vi "Car Wash Cycle.vi"(4 "Finish Message":string, 6 "Start Message":string, 7 "Time (ms)":u32=5000, 9 "Indicator":refnum<class "Abs_Boolean.lvclass">, 10 "Option":refnum<class "Abs_Boolean.lvclass">, 11 "EventLog":refnum<class "Event_TextLog.lvclass">) -> (3 "bt_Node out":refnum<class "bt_Node.lvclass">)   [LabVIEW 2021, in "Car Wash Support.lvlib"]
uses:
  Car Wash Support.lvlib
  <vilib>/TSA/Event Log/Event_TextLog/Event_TextLog.lvclass
  C:/Program Files (x86)/National Instruments/LabVIEW 2021/vi.lib/TSA/Event Log/abs_EventLog/abs_EventLog.lvclass
  <vilib>/TSA/Abstract Data Classes/Abs_Types/Boolean/Abs_Boolean.lvclass
  C:/Program Files (x86)/National Instruments/LabVIEW 2021/vi.lib/TSA/Abstract Data Classes/Abs_Types/Value/Abs_Value.lvclass
  C:/Program Files (x86)/National Instruments/LabVIEW 2021/vi.lib/TSA/Abstract Data Classes/Abs_Types/Type/Abs_Type.lvclass
  Support/Nodes/abs_Node/bt_Node.lvclass
  Support/Nodes/Leaves/abs_Type Leaf/abs_Type Leaf.lvclass/abs_Type Leaf.ctl
  Support/Nodes/Leaves/abs_Type Leaf/Properties/Write Value Class.vi
  Support/Nodes/Leaves/Test Boolean/Test Abs_Boolean.lvclass
  C:/Users/timst/Documents/Repositories/LV_Behaviour_Tree/Source/Support/Nodes/abs_Node/bt_Node.lvclass
  C:/Users/timst/Documents/Repositories/LV_Behaviour_Tree/Source/Support/Nodes/Leaves/abs_Type Leaf/abs_Type Leaf.lvclass
  Support/Nodes/Leaves/Log/bt_Log.lvclass
  <vilib>/TSA/Abstract Data Classes/Constants/Support/Bool/Bool.vi
  <vilib>/TSA/Abstract Data Classes/Constants/Support/Str/Str.vi
  Support/Poly/Log/Log_StringClass.vi
  BT.lvlib
  <vilib>/TSA/Abstract Data Classes/Constants/Support/Bool/Const_Bool.lvclass
  <vilib>/TSA/Abstract Data Classes/Constants/Support/Str/Const_Str.lvclass
  C:/Program Files (x86)/National Instruments/LabVIEW 2021/vi.lib/TSA/Event Log/Event_TextLog/Event_TextLog.lvclass
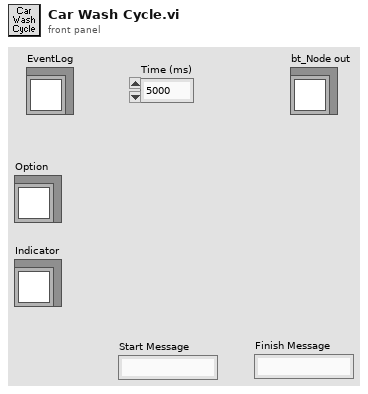
[diagram p1: front panel]
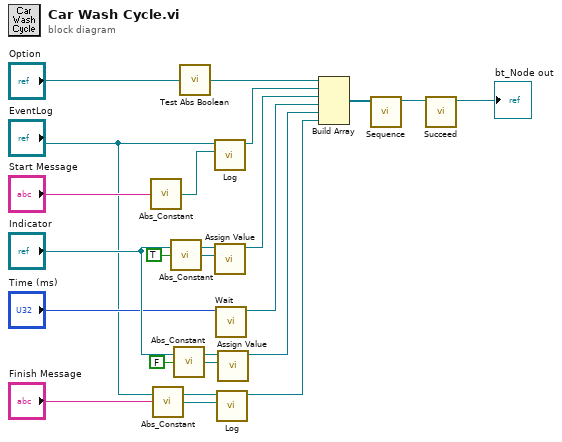
[diagram p0: block diagram]
diagram:
  n1 = call-poly <vilib>:"Abs_Constant.vi"("String"="Start Message") -> ("Abs_String.lvclass"=w16:refnum<class "Abs_String.lvclass">)  [unwired: 4 in]
  n2 = call-poly <vilib>:"Abs_Constant.vi"("String"="Finish Message") -> ("Abs_String.lvclass"=w19:refnum<class "Abs_String.lvclass">)  [unwired: 4 in]
  n3 = call-poly <vilib>:"Abs_Constant.vi"("Boolean"=TRUE) -> ("Abs_Boolean.lvclass"=w6:refnum<class "Abs_Boolean.lvclass">)  [unwired: 4 in]
  n4 = call-poly <vilib>:"Abs_Constant.vi"("Boolean"=FALSE) -> ("Abs_Boolean.lvclass"=w11:refnum<class "Abs_Boolean.lvclass">)  [unwired: 4 in]
  n5 = call "Test Abs Boolean.vi"("Abs_Boolean.lvclass"="Option") -> ("abs_Node"=w5:refnum<class "bt_Node.lvclass">)  [unwired: 4 in]
  n6 = call-poly "Log.vi"("Message"=w16, "EventLog"="EventLog") -> ("node out"=w18:refnum<class "bt_Log.lvclass">)  [unwired: 9 in]
  n7 = call "Assign Value.vi"("Assigned Value"=w6, "Value"="Indicator") -> ("Node Out"=w8:refnum<class "bt_Node.lvclass">)  [unwired: 9 in]
  n8 = call "Wait.vi"("Time (ms)"="Time (ms)") -> ("Node Out"=w9:refnum<class "bt_Node.lvclass">)  [unwired: 10 in]
  n9 = call-poly "Log.vi"("Message"=w19, "EventLog"="EventLog") -> ("node out"=w20:refnum<class "bt_Log.lvclass">)  [unwired: 9 in]
  n10 = call "Assign Value.vi"("Assigned Value"=w11, "Value"="Indicator") -> ("Node Out"=w12:refnum<class "bt_Node.lvclass">)  [unwired: 9 in]
  n11 = Build Array(w5, w18, w8, w9, w12, w20) -> (w4:refnum<class "bt_Node.lvclass">[])
  n12 = call "Sequence.vi"("Nodes"=w4) -> ("Node"=w13:refnum<class "bt_Node.lvclass">)  [unwired: 10 in]
  n13 = call "Succeed.vi"("Node In"=w13) -> ("Node"=→"bt_Node out":refnum<class "bt_Node.lvclass">)  [unwired: 10 in]
